vi "Center Point dx dy to Rect.vi"(8 "错误输入":errorcluster, 10 "Para":cluster{"dx":i16, "dy":i16}={"dx"=10, "dy"=4}, 11 "Center":T1) -> (0 "错误输出":errorcluster, 3 "Rect Point Array":T1[](array[typedef]))   [LabVIEW 2011, in "Basic Shape.lvlib"]
uses:
  Basic Shape.lvlib
  Point Custom Control.ctl
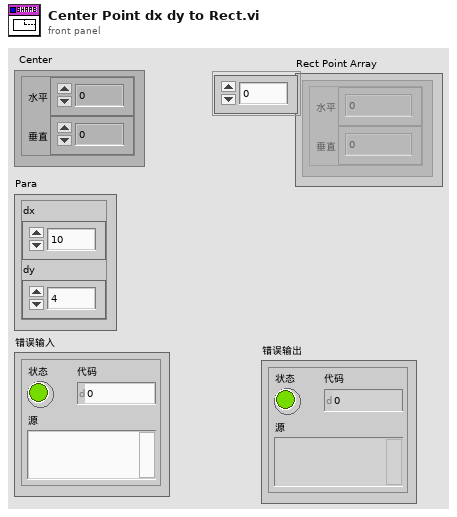
[diagram p1: front panel]
types:
  T1 = typedef "Basic Shape.lvlib/Point Custom Control.ctl" = cluster{"horizontal":i16, "vertical":i16}
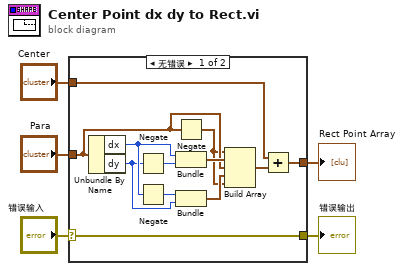
[diagram p0: block diagram]
diagram:
  n1 = case shown="无错误" "错误输入" {
    selector: "错误输入" -> [w17 w18]
    tunnel: [w17 w18] -> w4
    tunnel: "Para" -> [w11 _]
    tunnel: "Center" -> [w15 _]
    tunnel: [w14 _] -> w1
    frame No Error {
      n2 = Unbundle By Name(w11) -> ("dx"=w10:i16, "dy"=w8:i16)
      n3 = Negate(x=w8) -> (-x=w13:i16)
      n4 = Negate(x=w10) -> (-x=w9:i16)
      n5 = Negate(x=w11) -> (-x=w6:cluster{"dx":i16, "dy":i16})
      n6 = Bundle("dx"=w10, w13) -> (w12:cluster{"dx":i16, i16})  [unwired: 1 in]
      n7 = Bundle(w9, "dy"=w8) -> (w7:cluster{i16, "dy":i16})  [unwired: 1 in]
      n8 = Build Array(w6, w12, w11, w7, w6) -> (w16:cluster{"dx":i16, "dy":i16}[])
      n9 = Add(x=w15, y=w16) -> (x+y=w14:T1[])
    }
    frame Error {
    }
  }
  "错误输出" <- w4
  "Rect Point Array" <- w1
